vi "process_limits.vi"(10 "old output cluster":T1, 11 "Input cluster":T2) -> (0 "Update FPGA":bool, 3 "output cluster":T1)   [LabVIEW 2015]
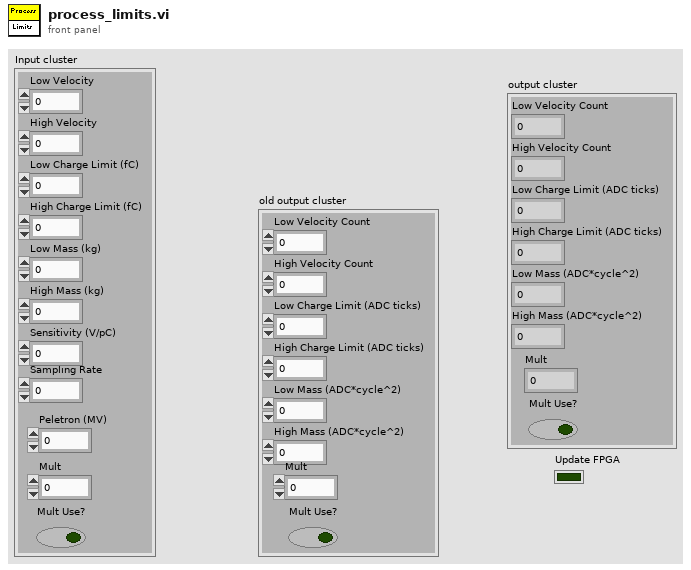
[diagram p1: front panel]
types:
  T1 = cluster{"Low Velocity Count":i32, "High Velocity Count":i32, "Low Charge Limit (ADC ticks)":i16, "High Charge Limit (ADC ticks)":i16, "Low Mass (ADC*cycle^2)":i64, "High Mass (ADC*cycle^2)":i64, "Mult":fxp<+,16,7>, "Mult Use?":bool}
  T2 = cluster{"Low Velocity":dbl, "High Velocity":dbl, "Low Charge Limit (fC)":dbl, "High Charge Limit (fC)":dbl, "Low Mass (kg)":dbl, "High Mass (kg)":dbl, "Sensitivity (V/pC)":dbl, "Sampling Rate":dbl, "Peletron (MV)":dbl, "Mult":fxp<+,16,7>, "Mult Use?":bool}
  T3 = cluster{"Low Velocity Count":i32, "High Velocity Count":i32, "Low Charge Limit (ADC ticks)":i16, "High Charge Limit (ADC ticks)":i16, "Low Mass (ADC*cycle^2)":i64, "High Mass (ADC*cycle^2)":i64}
  T4 = cluster{i32, i32, i16, i16, i64, i64, "Mult":fxp<+,16,7>, "Mult Use?":bool}
  T5 = cluster{"t":bool, "t":bool, "t":bool, "t":bool, "t":bool, "t":bool}
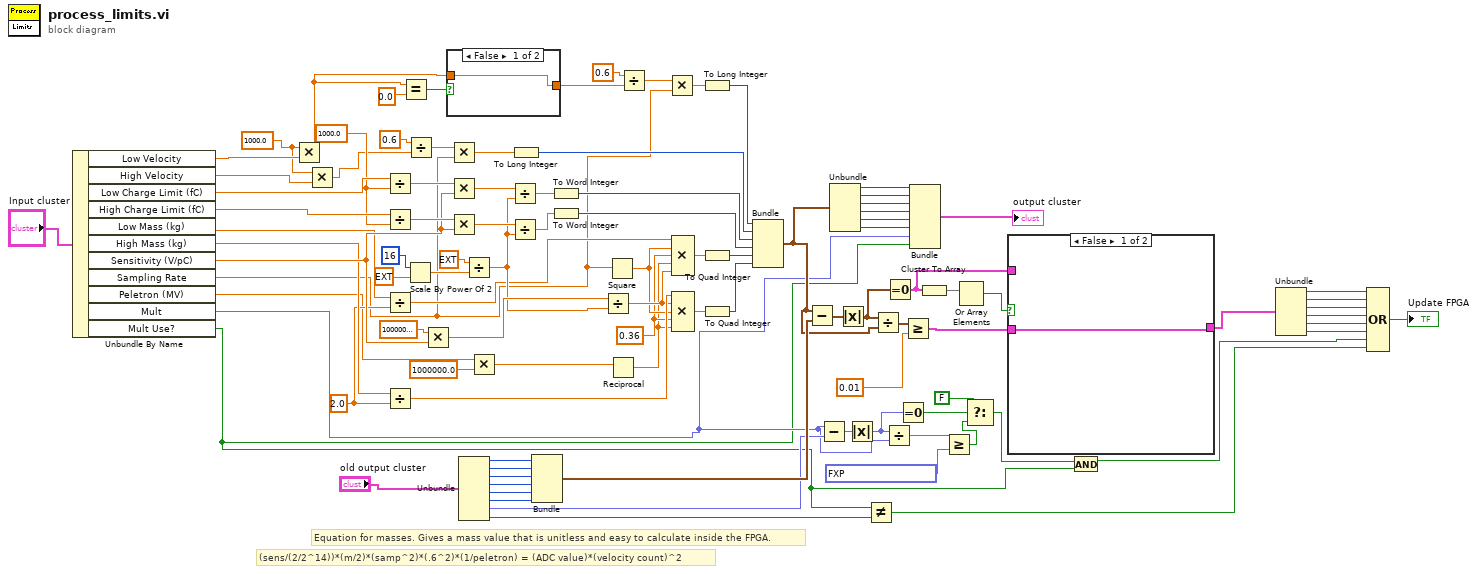
[diagram p0: block diagram]
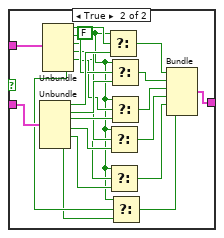
[diagram p2: hidden frame]
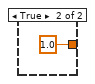
[diagram p3: hidden frame]
diagram:
  w49 = 1000.0 ("x")
  w58 = 0.36 ("value")
  w66 = 2.0 ("y")
  w79 = 1000.0 ("y")
  # "Equation for masses. Gives a mass value that is unitless and easy to calculate inside the FPGA."
  # "(sens/(2/2^14))*(m/2)*(samp^2)*(.6^2)*(1/peletron) = (ADC value)*(velocity count)^2"
  n1 = Unbundle By Name("Input cluster") -> ("Low Velocity"=w52:dbl, "High Velocity"=w50:dbl, "Low Charge Limit (fC)"=w87:dbl, "High Charge Limit (fC)"=w80:dbl, "Low Mass (kg)"=w68:dbl, "High Mass (kg)"=w67:dbl, "Sensitivity (V/pC)"=w72:dbl, "Sampling Rate"=w64:dbl, "Peletron (MV)"=w41:dbl, "Mult"=w20:fxp<+,16,7>, "Mult Use?"=w1:bool)
  n2 = Multiply(x=w49, y=w52) -> (x*y=w51:dbl)
  n3 = Multiply(x=w49, y=w50) -> (x*y=w48:dbl)
  n4 = Divide(x=w87, y=w79) -> (x/y=w86:dbl)
  n5 = Divide(x=w80, y=w79) -> (x/y=w78:dbl)
  n6 = Divide(x=w68, y=w66) -> (x/y=w65:dbl)
  n7 = Divide(x=w67, y=w66) -> (x/y=w61:dbl)
  n8 = Equal?(x=w51, y=0.0) -> (x = y?=w96:bool)
  n9 = Scale By Power Of 2(n=i16 16, x=ext 1.0) -> (x*2^n=w83:ext)
  n10 = Divide(x=0.6, y=w48) -> (x/y=w90:dbl)
  n11 = Multiply(x=1000000000000.0, y=w72) -> (x*y=w70:dbl)
  n12 = case shown="False" w96 {
    tunnel: [w100 1.0 ("y")] -> w95
    tunnel: w51 -> [w100 _]
    frame False {
    }
    frame True {
    }
  }
  n13 = Multiply(x=w90, y=w64) -> (x*y=w89:dbl)
  n14 = Multiply(x=w86, y=w72) -> (x*y=w77:dbl)
  n15 = Multiply(x=w78, y=w72) -> (x*y=w76:dbl)
  n16 = Unbundle("old output cluster") -> ("Low Velocity Count"=w37:i32, "High Velocity Count"=w36:i32, "Low Charge Limit (ADC ticks)"=w35:i16, "High Charge Limit (ADC ticks)"=w34:i16, "Low Mass (ADC*cycle^2)"=w33:i64, "High Mass (ADC*cycle^2)"=w32:i64, "Mult"=w22:fxp<+,16,7>, "Mult Use?"=w17:bool)
  n17 = Divide(x=ext 2.0, y=w83) -> (x/y=w69:ext)
  n18 = Multiply(x=w41, y=1000000.0) -> (x*y=w53:dbl)
  n19 = Divide(x=w77, y=w69) -> (x/y=w75:ext)
  n20 = Divide(x=w76, y=w69) -> (x/y=w74:ext)
  n21 = To Long Integer(number=w89) -> (32bit integer=w88:i32)
  n22 = Bundle("Low Velocity Count"=w37, "High Velocity Count"=w36, "Low Charge Limit (ADC ticks)"=w35, "High Charge Limit (ADC ticks)"=w34, "Low Mass (ADC*cycle^2)"=w33, "High Mass (ADC*cycle^2)"=w32) -> (w31:T3)  [unwired: 1 in]
  n23 = To Word Integer(number=w75) -> (16bit integer=w81:i16)
  n24 = To Word Integer(number=w74) -> (16bit integer=w73:i16)
  n25 = Divide(x=w70, y=w69) -> (x/y=w60:ext)
  n26 = Square(x=w64) -> (x^2=w59:dbl)
  n27 = Reciprocal(x=w53) -> (1/x=w57:dbl)
  n28 = Divide(x=0.6, y=w95) -> (x/y=w98:dbl)
  n29 = Multiply(x=w98, y=w64) -> (x*y=w93:dbl)
  n30 = Compound Arithmetic op=MULTIPLY(w65, w59, w58, w57, w60) -> (w63:ext)
  n31 = Compound Arithmetic op=MULTIPLY(w61, w60, w59, w58, w57) -> (w56:ext)
  n32 = To Long Integer(number=w93) -> (32bit integer=w92:i32)
  n33 = To Quad Integer(1:w63) -> (0:w62:i64)
  n34 = To Quad Integer(1:w56) -> (0:w55:i64)
  n35 = Bundle(w92, w88, w81, w73, w62, w55) -> (w30:cluster{i32, i32, i16, i16, i64, i64})  [unwired: 1 in]
  n36 = Subtract(x=w30, y=w31) -> (x-y=w40:cluster{i32, i32, i16, i16, i64, i64})
  n37 = Subtract(x=w20, y=w22) -> (x-y=w21:fxp<+/-,17,8>)
  n38 = Unbundle(w30) -> (w29:i32, w28:i32, w27:i16, w26:i16, w25:i64, w24:i64)
  n39 = Absolute Value(x=w40) -> (abs(x)=w4:cluster{i32, i32, i16, i16, i64, i64})
  n40 = Absolute Value(x=w21) -> (abs(x)=w11:fxp<+,16,7>)
  n41 = Not Equal?(x=w1, y=w17) -> (x != y?=w16:bool)
  n42 = Divide(x=w4, y=w30) -> (x/y=w3:cluster{dbl, dbl, dbl, dbl, dbl, dbl})
  n43 = Divide(x=w11, y=w20) -> (x/y=w19:fxp<+,32,16>)
  n44 = Equal To 0?(x=w4) -> (x = 0?=w5:cluster{bool, bool, bool, bool, bool, bool})
  n45 = Equal To 0?(x=w11) -> (x = 0?=w10:bool)
  n46 = Greater Or Equal?(x=w3, y=0.01) -> (x >= y?=w7:cluster{bool, bool, bool, bool, bool, bool})
  n47 = Bundle(w29, w28, w27, w26, w25, w24, "Mult"=w20, "Mult Use?"=w1) -> (→"output cluster":T4)  [unwired: 1 in]
  n48 = Cluster To Array(cluster=w5) -> (array=w9:bool[])
  n49 = Greater Or Equal?(x=w19, y=fxp<+,32,16> 0.0099945068359375) -> (x >= y?=w14:bool)
  n50 = Or Array Elements(Boolean array=w9) -> (logical OR=w8:bool)
  n51 = Select(t=FALSE, s=w10, f=w14) -> (s? t:f=w12:bool)
  n52 = case shown="False" w8 {
    tunnel: [w102 w103] -> w6
    tunnel: w7 -> [w102 w123]
    tunnel: w5 -> [_ w124]
    frame False {
    }
    frame True {
      w106 = FALSE ("t")
      n53 = Unbundle(w123) -> (w121:bool, w118:bool, w115:bool, w112:bool, w109:bool, w105:bool)
      n54 = Unbundle(w124) -> (w122:bool, w119:bool, w116:bool, w113:bool, w110:bool, w107:bool)
      n55 = Select(t=w106, s=w122, f=w121) -> (s? t:f=w120:bool)
      n56 = Select(t=w106, s=w113, f=w112) -> (s? t:f=w111:bool)
      n57 = Select(t=w106, s=w110, f=w109) -> (s? t:f=w108:bool)
      n58 = Select(t=w106, s=w119, f=w118) -> (s? t:f=w117:bool)
      n59 = Select(t=w106, s=w116, f=w115) -> (s? t:f=w114:bool)
      n60 = Select(t=w106, s=w107, f=w105) -> (s? t:f=w104:bool)
      n61 = Bundle("t"=w120, "t"=w117, "t"=w114, "t"=w111, "t"=w108, "t"=w104) -> (w103:T5)  [unwired: 1 in]
    }
  }
  n62 = And(x=w12, y=w1) -> (x .and. y?=w2:bool)
  n63 = Unbundle(w6) -> ("t"=w47:bool, "t"=w46:bool, "t"=w45:bool, "t"=w44:bool, "t"=w43:bool, "t"=w42:bool)
  n64 = Compound Arithmetic op=OR(w47, w46, w45, w44, w43, w42, w2, w16) -> (→"Update FPGA":bool)
